vi "SubVI1.vi"() -> ()   [LabVIEW 2018]
panel:
  out "Thermometer 2":dbl(slide) scale=0.0..100.0
  in  "OK Button":bool
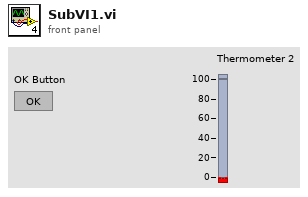
[diagram p1: front panel]
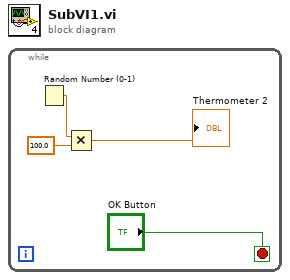
[diagram p0: block diagram]
diagram:
  n1 = while {
    stop <- "OK Button" stop-if-true
    n2 = Random Number (0-1)() -> (number: 0 to 1=w2:dbl)
    n3 = Multiply(x=w2, y=100.0) -> (x*y=→"Thermometer 2":dbl)
  }
